vi "Main.vi"() -> ()   [LabVIEW 2015, in "Thermometer.lvlib"]
doc: "This template is based off of the Queued Message Handler design pattern and the Queued Message Handler project template that ships with LabVIEW.\n\nThe main difference is that the queue is private to this module and communication between modules is performed via Broadcast and Request events.\n\nRequest events are wrapped in public API methods and are handled in the Event Handling Loop (EHL) of this VI. Any module can register for Broadcast events sent by this module. The EHL generates messages based on user interface actions.\n\nThe Message Handling Loop (MHL) processes messages generated by the EHL, or by other messages. The messages are string values, so new messages can be added easily to the Message Cases case structure in the MHL. Each message cluster can also provide an optional value for Message Data, which is a variant that can be converted to whatever message-specific data is required.\n_____\nBased on Delacor QMH Project Template 4.2.1.64."
uses:
  Thermometer.lvlib
  <vilib>/Delacor/Delacor QMH/Libraries/Module Admin_class/Delacor_lib_QMH_Module Admin.lvclass
  Module Data--cluster.ctl
  <vilib>/Delacor/Delacor QMH/Libraries/Message Queue_class/Delacor_lib_QMH_Message Queue.lvclass/Delacor_lib_QMH_Message Queue.ctl
  Stop Argument--cluster.ctl
  <vilib>/Delacor/Delacor QMH/Libraries/Module Admin_class/Delacor_lib_QMH_Module Admin.lvclass/Delacor_lib_QMH_Module Admin.ctl
  Start Argument--cluster.ctl
  <vilib>/Utility/miscctls.llb/LVPointTypeDef.ctl
  <vilib>/Delacor/Delacor QMH/Libraries/Message Queue_class/Delacor_lib_QMH_Enqueue Message (Single).vi
  <vilib>/Delacor/Delacor QMH/Libraries/Module Admin_class/Delacor_lib_QMH_Get External Launch.vi
  <vilib>/Utility/error.llb/Error Cluster From Error Code.vi
  <vilib>/ErrorRing/Error Ring.xnode
  <vilib>/Delacor/Delacor QMH/Libraries/Message Queue_class/Delacor_lib_QMH_Message Queue.lvclass
  <vilib>/measure/NI_MABase.lvlib
panel:
  out "Thermometer":dbl(slide) scale=0.0..100.0
  in  "Simulate MHL Error":bool
  in  "Simulate EHL Error":bool
  out "error out":errorcluster
  in  "Module Admin":refnum<class "Delacor_lib_QMH_Module Admin.lvclass">
  out "Status":string
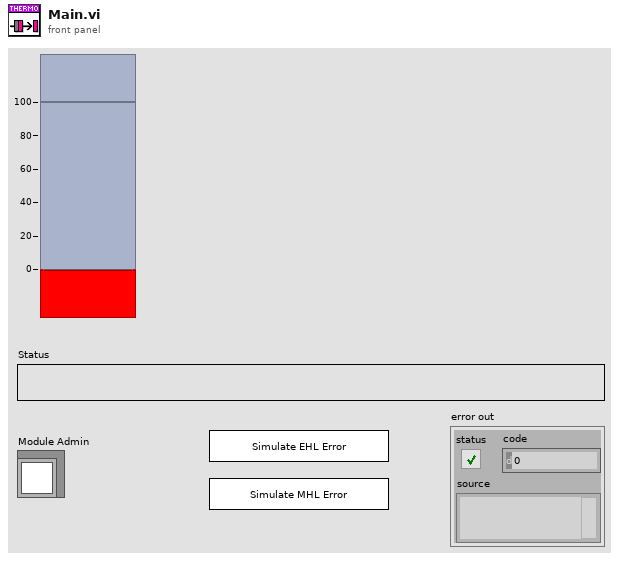
[diagram p1: front panel]
types:
  T1 = typedef "Thermometer.lvlib/Request Events--cluster.ctl" = cluster{"Stop Module":refnum<user-event>, "Show Panel":refnum<user-event>, "Hide Panel":refnum<user-event>, "Get Module Execution Status":refnum<user-event>, "Show Diagram":refnum<user-event>, "Start":refnum<user-event>}
  T2 = typedef "Thermometer.lvlib/Module Data--cluster.ctl" = cluster{"Status":string}
  T3 = enum16{"Sine Wave", "Triangle Wave", "Square Wave", "Sawtooth Wave"}
  T4 = enum32{"invalid lock state", "Not Locked", "Locked (No Password)", "Password-protected"}
  T5 = typedef "Thermometer.lvlib/Stop Argument--cluster.ctl" = cluster{"Origin":string, "Exit via Stop Module Req?":bool, "Wait for Module to stop?":bool}
  T6 = typedef "Thermometer.lvlib/Start Argument--cluster.ctl" = cluster{"Starting Temperature":dbl}
  T7 = typedef "LVPointTypeDef.ctl" = cluster{"Horizontal":i16, "Vertical":i16}
  T8 = enum32{"Invalid", "Standard", "Closed", "Hidden", "Minimized", "Maximized"}
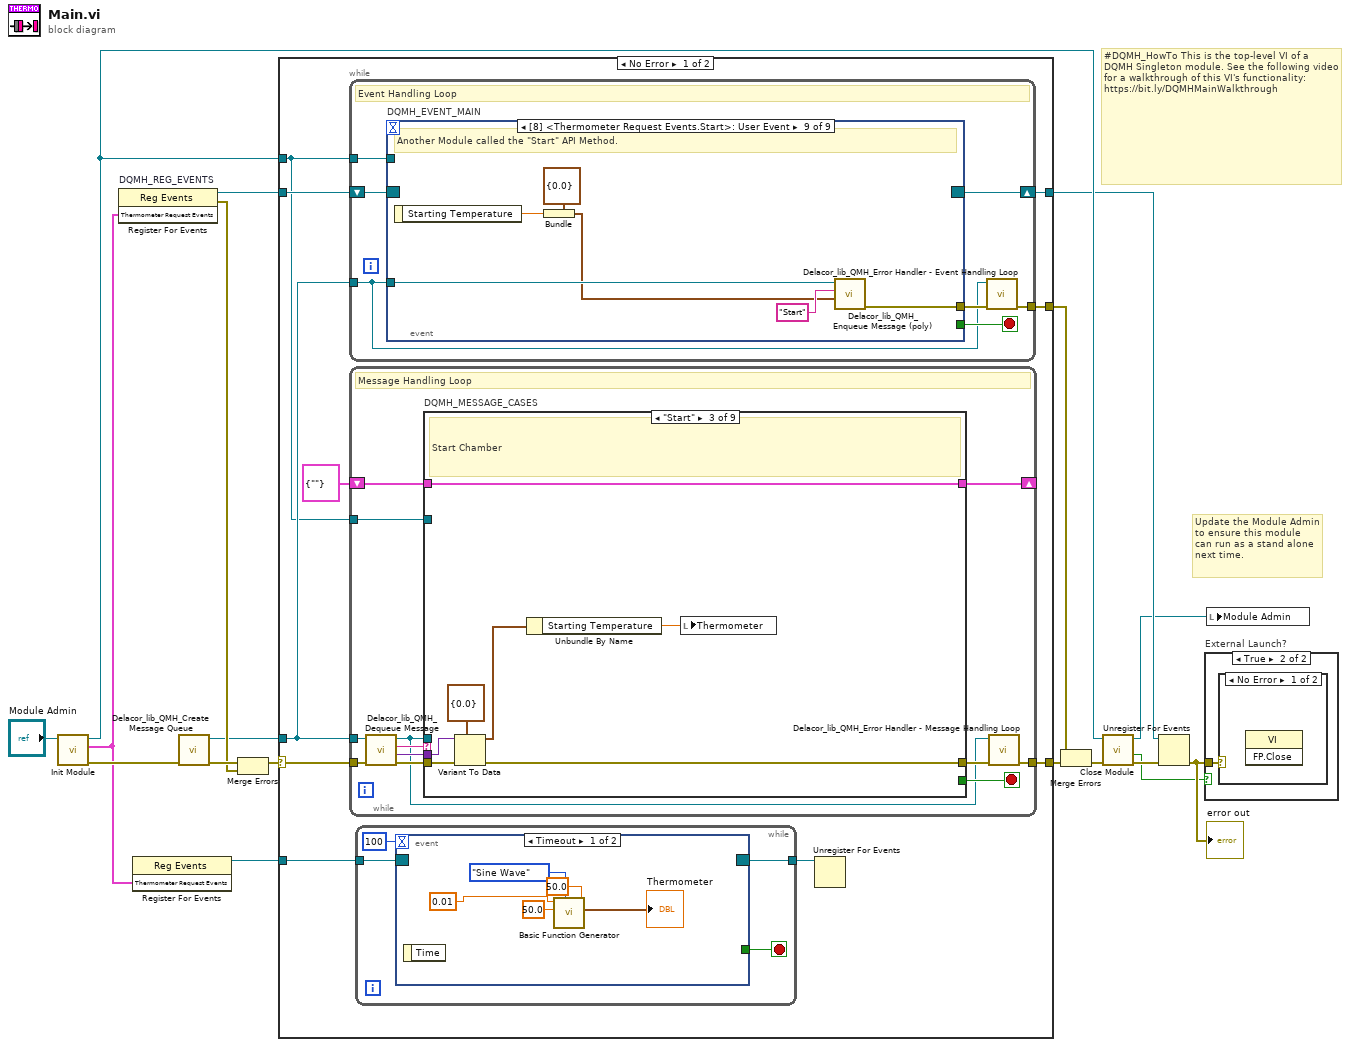
[diagram p0: block diagram]
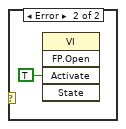
[diagram p3: hidden frame]
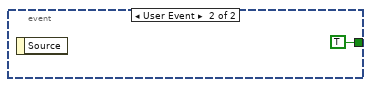
[diagram p4: hidden frame]
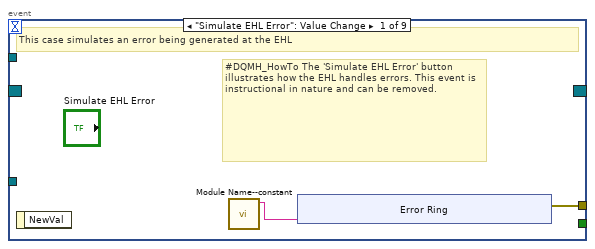
[diagram p5: hidden frame]
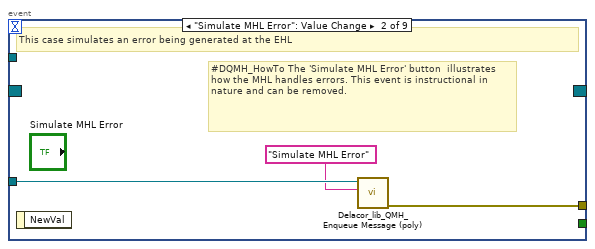
[diagram p6: hidden frame]
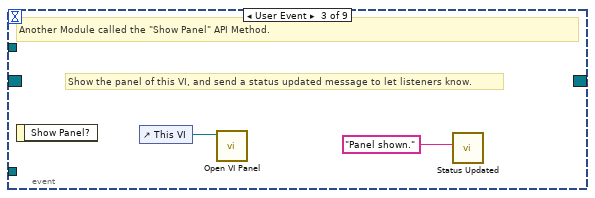
[diagram p7: hidden frame]
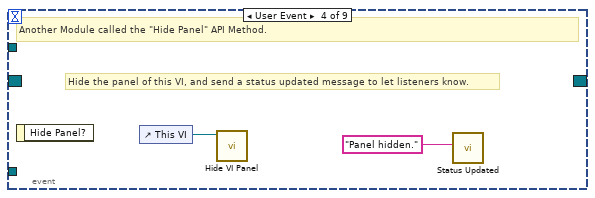
[diagram p8: hidden frame]
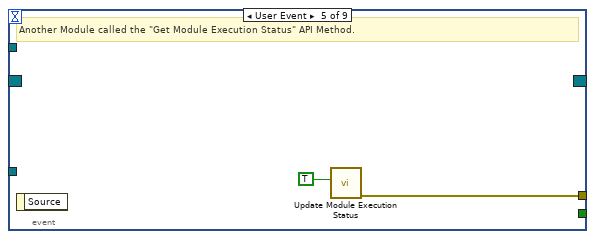
[diagram p9: hidden frame]
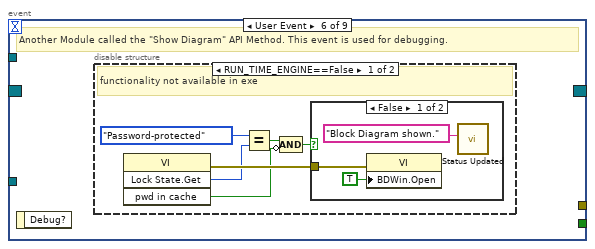
[diagram p10: hidden frame]
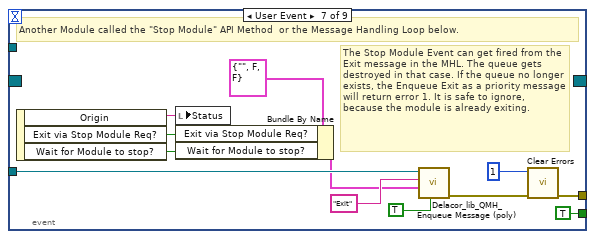
[diagram p13: hidden frame]
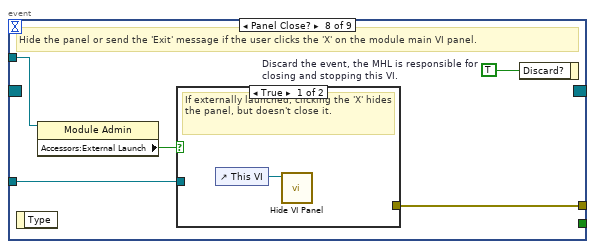
[diagram p14: hidden frame]
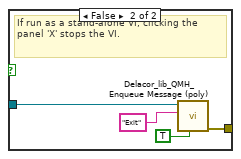
[diagram p15: hidden frame]
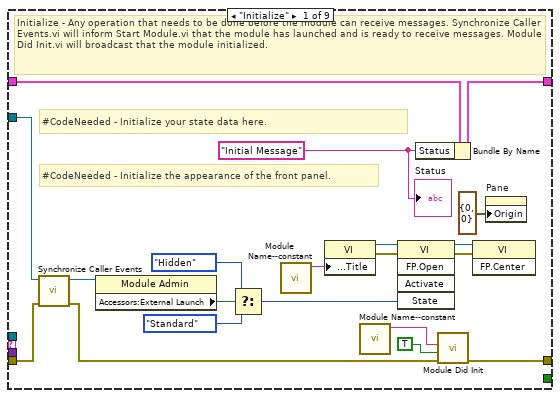
[diagram p16: hidden frame]
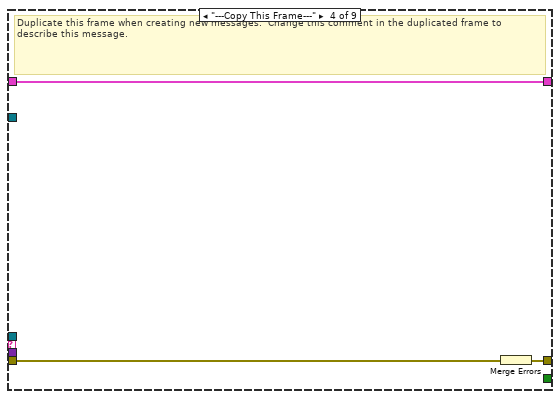
[diagram p18: hidden frame]
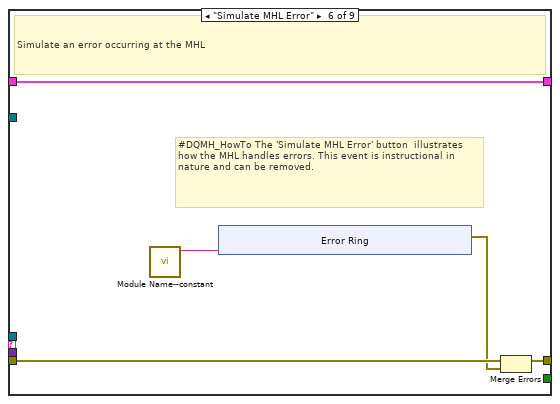
[diagram p20: hidden frame]
diagram:
  # "#DQMH_HowTo This is the top-level VI of a DQMH Singleton module. See the following video for a walkthrough of this VI's functionality: https://bit.ly/DQMHMainWalkthrough"
  # "Update the Module Admin to ensure this module can run as a stand alone next time."
  n1 = call "Init Module.vi"("Singleton Module Admin in"="Module Admin") -> ("error out"=w17:errorcluster, "Thermometer Request Events"=w2:T1, "Singleton Module Admin out"=w9:refnum<class "Delacor_lib_QMH_Module Admin.lvclass">)  [unwired: 8 in]
  n2 = register-events "DQMH_REG_EVENTS"(w2) -> (reference out=w7:refnum<event-registration>, error out=w10:errorcluster)  [unwired: 2 in]
  n3 = register-events(w2) -> (reference out=w1:refnum<event-registration>)  [unwired: 2 in, 1 out]
  n4 = call <vilib>:"Delacor_lib_QMH_Create Message Queue.vi"("error in (no error)"=w17) -> ("error out"=w12:errorcluster, "Message Queue"=w6:refnum<class "Delacor_lib_QMH_Message Queue.lvclass">)  [unwired: 9 in]
  n5 = Merge Errors(w12, w10) -> (w11:errorcluster)
  n6 = case shown="No Error" w11 {
    selector: w11 -> [w26 w211]
    tunnel: [w28 w211] -> w18
    tunnel: [w25 w208] -> w8
    tunnel: w7 -> [w23 w208]
    tunnel: w6 -> [w22 _]
    tunnel: [w27 _] -> w15
    tunnel: w9 -> [w21 w204]
    tunnel: w1 -> [w20 _]
    frame No Error {
      n7 = while {
        tunnel: w22 -> [w39]
        shift-right: [w42] -> w25
        shift-left: w23 -> [w43]
        tunnel: [w44] -> w27
        tunnel: w21 -> [w40]
        stop <- w41 stop-if-true
        # "Event Handling Loop"
        n8 = event "DQMH_EVENT_MAIN" shown="[8] <Thermometer Request Events.Start>: User Event" {
          selector: w43 -> [_ _ _ _ _ _ _ _ _]
          dyn-events: [_ _ _ _ _ _ _ _ _] -> w42
          timeout: _ -> [_ _ _ _ _ _ _ _ _]
          tunnel: [_ _ _ _ _ _ TRUE ("Discard?") _ _] -> w41
          tunnel: w39 -> [_ w56 _ _ _ _ w80 w87 w100]
          tunnel: [w47 w57 _ _ w63 _ w83 w89 w96] -> w45
          tunnel: w40 -> [_ _ _ _ _ _ _ w86 _]
          event "Simulate EHL Error": Value Change {
            # "#DQMH_HowTo The 'Simulate EHL Error' button  illustrates how the EHL handles errors. This event is instructional in nature and can be removed."
            # "This case simulates an error being generated at the EHL"
            n9 = event-data() -> ()  [unwired: 1 in, 1 out]
            n10 = call "Module Name--constant.vi"() -> ("Module Name"=w46:string)  [unwired: 11 in]
            n11 = xnode "Error Ring"("parameter 0"=w46) -> ("error out"=w47:errorcluster)
          }
          event "Simulate MHL Error": Value Change {
            # "#DQMH_HowTo The 'Simulate MHL Error' button  illustrates how the MHL handles errors. This event is instructional in nature and can be removed."
            # "This case simulates an error being generated at the EHL"
            n12 = event-data() -> ()  [unwired: 1 in, 1 out]
            n13 = call-poly <vilib>:"Delacor_lib_QMH_Enqueue Message (poly).vi"("Message"="Simulate MHL Error", "Message Queue in"=w56) -> ("error out"=w57:errorcluster)  [unwired: 8 in, 1 out]
          }
          event User Event {
            # "Show the panel of this VI, and send a status updated message to let listeners know."
            # "Another Module called the \"Show Panel\" API Method."
            n14 = event-data() -> ()  [unwired: 1 in, 1 out]
            n15 = control-ref of="This VI"() -> (w59:refnum<vi>)
            n16 = call "Open VI Panel.vi"("VI"=w59) -> ()  [unwired: 10 in, 1 out]
            n17 = call "Status Updated.vi"("Status"="Panel shown." ("format string")) -> ()  [unwired: 10 in, 1 out]
          }
          event User Event {
            # "Hide the panel of this VI, and send a status updated message to let listeners know."
            # "Another Module called the \"Hide Panel\" API Method."
            n18 = event-data() -> ()  [unwired: 1 in, 1 out]
            n19 = control-ref of="This VI"() -> (w61:refnum<vi>)
            n20 = call "Hide VI Panel.vi"("VI"=w61) -> ()  [unwired: 10 in, 1 out]
            n21 = call "Status Updated.vi"("Status"="Panel hidden." ("format string")) -> ()  [unwired: 10 in, 1 out]
          }
          event User Event {
            # "Another Module called the \"Get Module Execution Status\" API Method."
            n22 = event-data() -> ()  [unwired: 1 in, 1 out]
            n23 = call "Update Module Execution Status.vi"("Running?"=TRUE) -> ("error out"=w63:errorcluster)  [unwired: 10 in]
          }
          event User Event {
            # "Another Module called the \"Show Diagram\" API Method. This event is used for debugging."
            n24 = event-data() -> ()  [unwired: 1 in, 1 out]
            n25 = disable-structure shown="RUN_TIME_ENGINE==False" {
              frame condition #0 (active) {
                # "functionality not available in exe"
                n26 = invoke class="VI" method="Lock State.Get"() -> (error out=w69:errorcluster, "Get Lock State"=w68:T4, "pwd in cache"=w65:bool)  [unwired: 4 in, 1 out]
                n27 = Equal?(x=T4."Password-protected", y=w68) -> (x = y?=w66:bool)
                n28 = Compound Arithmetic op=AND(w66, invert w65) -> (w64:bool)
                n29 = case shown="False" w64 {
                  tunnel: w69 -> [w72 _]
                  frame False {
                    n30 = property class="VI"(error in=w72, "BDWin.Open"=TRUE ("Block Diagram Window:Open")) -> ()  [unwired: 1 in, 2 out]
                    n31 = call "Status Updated.vi"("Status"="Block Diagram shown." ("format string")) -> ()  [unwired: 10 in, 1 out]
                  }
                  frame True {
                    # "Password-protected VI, and the password is not in the cache. Do not show the diagram."
                  }
                }
              }
              frame condition #1 {
              }
            }
          }
          event User Event {
            # "The Stop Module Event can get fired from the Exit message in the MHL. The queue gets destroyed in that case. If the queue no longer exists, the Enqueue Exit as a priority message will return error 1. It is safe to ignore, because the module is already exiting."
            # "Another Module called the \"Stop Module\" API Method  or the Message Handling Loop below."
            n32 = event-data() -> ("Origin"=w79:string, "Exit via Stop Module Req?"=w75:bool, "Wait for Module to stop?"=w74:bool)  [unwired: 1 in]
            n33 = local write "Status"(w79) -> ()
            n34 = Bundle By Name(cluster=T5 {"Origin"="", "Exit via Stop Module Req?"=FALSE, "Wait for Module to stop?"=FALSE} ("Stop Argument"), "Exit via Stop Module Req?"=w75, "Wait for Module to stop?"=w74) -> (w73:T5)
            n35 = call-poly <vilib>:"Delacor_lib_QMH_Enqueue Message (poly).vi"("Priority Message? (F)"=TRUE, "Message Data"=w73, "Message"="Exit", "Message Queue in"=w80) -> ("error out"=w84:errorcluster)  [unwired: 6 in, 1 out]
            n36 = call <vilib>:"Clear Errors.vi"("error in (no error)"=w84, "specific error code to clear (0: all)"=1) -> ("error out"=w83:errorcluster)  [unwired: 4 in, 1 out]
          }
          event Panel Close? {
            w88 = TRUE  # Discard the event, the MHL is responsible for closing and stopping this VI.
            # "Hide the panel or send the 'Exit' message if the user clicks the 'X' on the module main VI panel."
            n37 = event-data() -> ()  [unwired: 1 in, 1 out]
            n38 = property class="Module Admin"(reference=w86) -> ("Accessors:External Launch"=w85:bool)  [unwired: 1 in, 2 out]
            n39 = case shown="True" w85 {
              tunnel: w87 -> [_ w93]
              tunnel: [_ w94] -> w89
              frame True {
                # "If externally launched, clicking the 'X' hides the panel, but doesn't close it."
                n40 = control-ref of="This VI"() -> (w90:refnum<vi>)
                n41 = call "Hide VI Panel.vi"("VI"=w90) -> ()  [unwired: 10 in, 1 out]
              }
              frame False {
                # "If run as a stand-alone VI, clicking the panel 'X' stops the VI."
                n42 = call-poly <vilib>:"Delacor_lib_QMH_Enqueue Message (poly).vi"("Priority Message? (F)"=TRUE, "Message"="Exit", "Message Queue in"=w93) -> ("error out"=w94:errorcluster)  [unwired: 7 in, 1 out]
              }
            }
            n43 = event-data("Discard?"=w88) -> ()  [unwired: 1 in, 1 out]
          }
          event User Event {
            # "Another Module called the \"Start\" API Method."
            n44 = event-data() -> ("Starting Temperature"=w95:dbl)  [unwired: 1 in]
            n45 = Bundle(cluster=T6 {"Starting Temperature"=0.0} ("Start Argument"), "Starting Temperature"=w95) -> (w97:T6)
            n46 = call-poly <vilib>:"Delacor_lib_QMH_Enqueue Message (poly).vi"("Message Data"=w97, "Message"="Start", "Message Queue in"=w100) -> ("error out"=w96:errorcluster)  [unwired: 7 in, 1 out]
          }
        }
        n47 = call-dynamic "Delacor_lib_QMH_Error Handler - Event Handling Loop.vi"("error in (no error)"=w45, "Message Queue in"=w39) -> ("dup error in"=w44:errorcluster)  [unwired: 8 in, 1 out]
      }
      n48 = while {
        tunnel: w22 -> [w103]
        shift-right: [w107] -> _
        shift-left: T2 {"Status"=""} ("Data Cluster") -> [w108]
        tunnel: w26 -> [w111]
        tunnel: [w109] -> w28
        tunnel: w21 -> [w101]
        stop <- w106 stop-if-true
        # "Message Handling Loop"
        n49 = call-dynamic "Delacor_lib_QMH_Dequeue Message.vi"("error in (no error)"=w111, "Message Queue in"=w103) -> ("error out"=w110:errorcluster, "Message Data"=w104:variant, "Message"=w105:string, "Message Queue out"=w102:refnum<class "Delacor_lib_QMH_Message Queue.lvclass">)  [unwired: 6 in]
        n50 = case "DQMH_MESSAGE_CASES" shown="\"Start\"" w105 {
          selector: w105 -> [_ _ _ _ _ _ _ _ w191]
          tunnel: w102 -> [_ _ _ _ _ _ w161 w183 _]
          tunnel: w110 -> [w130 w134 w141 w144 w146 w151 w168 w189 w193]
          tunnel: [w128 w134 w139 w143 w146 w150 w164 w186 w194] -> w112
          tunnel: w108 -> [w119 w133 w140 w142 w145 w148 w163 w182 w192]
          tunnel: [w118 w133 w140 w142 w145 w148 w163 w182 w192] -> w107
          tunnel: [_ _ _ _ _ _ _ w181 _] -> w106
          tunnel: w104 -> [_ _ w138 _ _ _ w162 w180 _]
          tunnel: w101 -> [w120 _ _ _ _ _ w160 w175 _]
          frame "Initialize" {
            w113 = "Initial Message" ("Initial Message")
            # "#CodeNeeded - Initialize the appearance of the front panel."
            # "#CodeNeeded - Initialize your state data here."
            # "Initialize - Any operation that needs to be done before the module can receive messages. Synchronize Caller Events.vi will inform Start Module.vi that the module has launched and is ready to receive messages. Module Did Init.vi will broadcast that the module initialized."
            n51 = call "Synchronize Caller Events.vi"("error in (no error)"=w130, "Singleton Module Admin in"=w120) -> ("error out"=w129:errorcluster, "Singleton Module Admin out"=w115:refnum<class "Delacor_lib_QMH_Module Admin.lvclass">)  [unwired: 8 in]
            n52 = property class="Module Admin"(reference=w115) -> ("Accessors:External Launch"=w124:bool)  [unwired: 1 in, 2 out]
            n53 = Select(t=T8."Hidden" ("State"), s=w124, f=T8."Standard" ("State")) -> (s? t:f=w121:T8)
            n54 = call "Module Name--constant.vi"() -> ("Module Name"=w127:string)  [unwired: 11 in]
            n55 = property class="VI"("Front Panel.Title"=w127) -> (reference out=w126:refnum<vi>, error out=w132:errorcluster)  [unwired: 2 in]
            n56 = call "Module Name--constant.vi"() -> ("Module Name"=w116:string)  [unwired: 11 in]
            n57 = invoke class="VI" method="FP.Open"(reference=w126, error in=w132, "State"=w121) -> (reference out=w125:refnum<vi>, error out=w131:errorcluster)  [unwired: 2 in, 3 out]
            n58 = Bundle By Name(cluster=w119, "Status"=w113) -> (w118:T2)
            n59 = call "Module Did Init.vi"("error in (no error)"=w129, "Initialized?"=TRUE, "Origin"=w116) -> ("error out"=w128:errorcluster)  [unwired: 8 in]
            n60 = invoke class="VI" method="FP.Center"(reference=w125, error in=w131) -> ()  [unwired: 1 in, 3 out]
            n61 = property on="Pane" class="Pane"("Origin"=T7 {"Horizontal"=0, "Vertical"=0}) -> ()  [unwired: 2 in, 2 out]
            "Status" <- w113
          }
          frame "--- Module Specific ---" {
            # "Separator -- The following cases handle messages specific to this Module."
          }
          frame "Start" {
            # "Start Chamber"
            n62 = Variant To Data(error in=w141, type=T6 {"Starting Temperature"=0.0} ("Start Argument"), Variant=w138) -> (data=w136:T6, error out=w139:errorcluster)
            n63 = Unbundle By Name(w136) -> ("Starting Temperature"=w135:dbl)
            n64 = local write "Thermometer"(w135) -> ()
          }
          frame "---Copy This Frame---" {
            # "Duplicate this frame when creating new messages.  Change this comment in the duplicated frame to describe this message."
            n65 = Merge Errors(w144) -> (w143:errorcluster)
          }
          frame "--- Exit and Error Handling---" {
            # "Separator - The following cases handle errors and exit messages."
          }
          frame "Simulate MHL Error" {
            # "#DQMH_HowTo The 'Simulate MHL Error' button  illustrates how the MHL handles errors. This event is instructional in nature and can be removed."
            # "Simulate an error occurring at the MHL"
            n66 = call "Module Name--constant.vi"() -> ("Module Name"=w147:string)  [unwired: 11 in]
            n67 = xnode "Error Ring"("parameter 0"=w147) -> ("error out"=w149:errorcluster)
            n68 = Merge Errors(w151, w149) -> (w150:errorcluster)
          }
          frame "Error" {
            # "#CodeRecommended - If you ever change the name of this \"Error\" message, you'll need to update the name in the Check Loop Error.vi as well."
            # "#CodeRecommended - If the module is running in standalone mode (External Launch = FALSE), this code will pop up an error dialog and call the 'Exit' message if an error occurs. Add more fine-grained error handling here."
            # "Error - Check the error message data and respond accordingly. This message is sent by the \"Error Handler\" VIs at the end of each loop in this application."
            n69 = property class="Module Admin"(reference=w160) -> ("Accessors:External Launch"=w159:bool)  [unwired: 1 in, 2 out]
            n70 = Variant To Data(error in=w168, type=errorcluster {"status"=FALSE, "code"=0, "source"=""} ("error constant"), Variant=w162) -> (data=w169:errorcluster, error out=w166:errorcluster)
            n71 = call "Error Reported.vi"("Error"=w169) -> ()  [unwired: 10 in, 1 out]
            n72 = case shown="False" w159 {
              tunnel: [w174 _] -> w165
              tunnel: w161 -> [w172 _]
              tunnel: w169 -> [w173 _]
              frame False {
                # "If the module is running standalone, then pop up an error dialog and call the \"Exit\" message."
                n73 = call <vilib>:"Simple Error Handler.vi"("error in (no error)"=w173) -> ()  [unwired: 4 in, 5 out]
                n74 = call-poly <vilib>:"Delacor_lib_QMH_Enqueue Message (poly).vi"("Priority Message? (F)"=TRUE, "Message"="Exit", "Message Queue in"=w172) -> ("error out"=w174:errorcluster)  [unwired: 7 in, 1 out]
              }
              frame True {
                # "If the module was launched externally, calling the Error Reported broadcast VI is the only action performed by the \"Error\" message. The module's caller can then process the error appropriately."
              }
            }
            n75 = Merge Errors(w166, w165) -> (w164:errorcluster)
            n76 = local write "error out"(w164) -> ()
          }
          frame "Exit" {
            w179 = 91  # 91: not all Exit messages will have an argument
            w181 = TRUE  # Stop the VI
            # "Release the message queue reference"
            # "#CodeNeeded - Add any required cleanup code here"
            # "Exit - Exit the application."
            n77 = Variant To Data(error in=w189, type=T5 {"Origin"="", "Exit via Stop Module Req?"=FALSE, "Wait for Module to stop?"=FALSE} ("Stop Argument"), Variant=w180) -> (data=w177:T5, error out=w185:errorcluster)
            n78 = call <vilib>:"Clear Errors.vi"("error in (no error)"=w185, "specific error code to clear (0: all)"=w179) -> ("error out"=w188:errorcluster)  [unwired: 4 in, 1 out]
            n79 = control-ref of="This VI"() -> (w176:refnum<vi>)
            n80 = call-dynamic "Delacor_lib_QMH_Release Message Queue.vi"("error in (no error)"=w188, "Message Queue"=w183) -> ("error out"=w187:errorcluster)  [unwired: 9 in]
            n81 = call "Handle Exit.vi"("Stop Argument"=w177, "Admin in"=w175, "VI reference"=w176) -> ("error out"=w184:errorcluster)  [unwired: 7 in, 1 out]
            n82 = Merge Errors(w187, w184) -> (w186:errorcluster)
          }
          frame Default {
            # "'Default' case only runs if there is a message that isn't defined in any of the other cases.  Output a programming error."
            n83 = call "Module Name--constant.vi"() -> ("Module Name"=w190:string)  [unwired: 11 in]
            n84 = xnode "Error Ring"("parameter 0"=w191, "parameter 1"=w190) -> ("error out"=w195:errorcluster)
            n85 = Merge Errors(w193, w195) -> (w194:errorcluster)
          }
        }
        n86 = call-dynamic "Delacor_lib_QMH_Error Handler - Message Handling Loop.vi"("error in (no error)"=w112, "Message Queue in"=w102) -> ("dup error in"=w109:errorcluster)  [unwired: 8 in, 1 out]
      }
      n87 = while {
        tunnel: w20 -> [w31]
        tunnel: [w30] -> w19
        stop <- w29 stop-if-true
        n88 = event shown="[0] Timeout" {
          selector: w31 -> [_ _]
          dyn-events: [_ _] -> w30
          timeout: 100 -> [_ _]
          tunnel: [_ TRUE] -> w29
          event Timeout {
            n89 = event-data() -> ()  [unwired: 1 in, 1 out]
            n90 = call <vilib>:"Basic Function Generator.vi"("offset"=50.0, "signal type"=T3."Sine Wave", "amplitude"=50.0, "frequency"=0.01) -> ("signal out"=→"Thermometer":waveform(dbl))  [unwired: 5 in, 2 out]
          }
          event User Event {
            n91 = event-data() -> ()  [unwired: 1 in, 1 out]
          }
        }
      }
      n92 = Unregister For Events(event registration refnum=w19) -> ()  [unwired: 1 in, 1 out]
    }
    frame Error {
      # "Synchronize Caller Events.vi will inform Start Module.vi that the module has launched and will let the code calling Start Module.vi register for broadcasts and would permit the caller receive the broadcast that an error occurred at launch time."
      n93 = call "Synchronize Caller Events.vi"("Singleton Module Admin in"=w204) -> ("error out"=w209:errorcluster)  [unwired: 9 in, 1 out]
      n94 = call "Module Name--constant.vi"() -> ("Module Name"=w207:string)  [unwired: 11 in]
      n95 = Format Into String(format string="An error occurred during initialization. %s is no longer running.", w207) -> (resulting string=w205:string)  [unwired: 2 in, 1 out]
      n96 = Merge Errors(w211, w209) -> (w210:errorcluster)
      n97 = call "Error Reported.vi"("Additional Information"=w205, "Error"=w210) -> ()  [unwired: 9 in, 1 out]
    }
  }
  n98 = Merge Errors(w15, w18) -> (w14:errorcluster)
  n99 = call "Close Module.vi"("error in (no error)"=w14, "Module Admin in"=w9) -> ("error out"=w16:errorcluster, "External Launch"=w3:bool, "Module Admin out"=w4:refnum<class "Delacor_lib_QMH_Module Admin.lvclass">)  [unwired: 7 in]
  n100 = Unregister For Events(event registration refnum=w8, error in=w16) -> (error out=w13:errorcluster)
  "error out" <- w13
  n101 = case "External Launch?" shown="True" w3 {
    tunnel: w13 -> [_ w212]
    frame False {
    }
    frame True {
      n102 = case shown="No Error" w212 {
        frame No Error {
          n103 = invoke class="VI" method="FP.Close"() -> ()  [unwired: 3 in, 3 out]
        }
        frame Error {
          n104 = invoke class="VI" method="FP.Open"("Activate"=TRUE ("Activate?")) -> ()  [unwired: 4 in, 5 out]
        }
      }
    }
  }
  n105 = local write "Module Admin"(w4) -> ()
